vi "Test_IncrementValuePublication_String_ErrorReturned.vi"(8 "error in (no error)":errorcluster, 11 "TestCase in":refnum<class "TestPublicationPolicy.lvclass">) -> (0 "error out":errorcluster, 3 "TestCase out":refnum<class "TestPublicationPolicy.lvclass">)   [LabVIEW 2017, in "TestPublicationPolicy.lvclass"]
uses:
  TestPublicationPolicy.lvclass
  Source/Framework/PublicationPolicy/IncrementValuePublication/IncrementValuePublication.lvclass
  C:/Git/mva-framework/Source/Framework/IMediator/IPublicationPolicy/IPublicationPolicy.lvclass
  Source/Framework/IMediator/IPublicationPolicy/IPublicationPolicy.lvclass
  gpm_packages/@cs/transport/Source/Concrete/NotifierTransport/NotifierTransport.lvclass/NotifierTransport.ctl
  Source/Framework/IMediator/PublishRequest/PublishRequest.lvclass/PublishRequest.ctl
  Source/Framework/IMediator/MutexedPublishRequest/MutexedPublishRequest.lvclass/MutexedPublishRequest.ctl
  Source/Framework/IMediator/PublishRequest/Write Publish Request Data.vi
  gpm_packages/@cs/transport/Source/Concrete/NotifierTransport/NotifierTransport.lvclass
  C:/Git/mva-framework/gpm_packages/@cs/transport/Source/ITransport/ITransport.lvclass
  Source/Framework/IMediator/MutexedPublishRequest/MutexedPublishRequest.lvclass
  C:/Git/mva-framework/Source/Framework/IMediator/PublishRequest/PublishRequest.lvclass
  <vilib>/Utility/error.llb/Error Cluster From Error Code.vi
panel:
  out "Publish Return Error":errorcluster
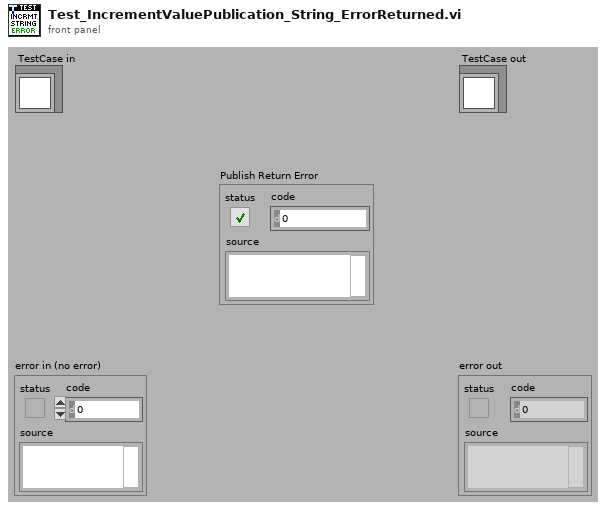
[diagram p1: front panel]
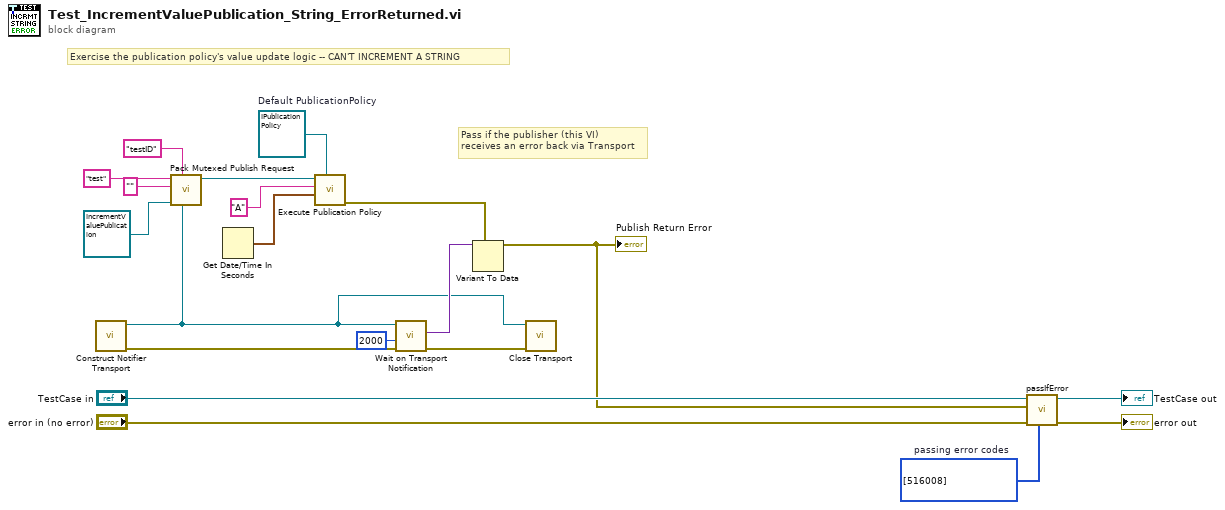
[diagram p0: block diagram]
diagram:
  w3 = i32[] [516008]  # passing error codes
  w12 = refnum<class "IPublicationPolicy.lvclass"> refnum  # Default PublicationPolicy
  # "Pass if the publisher (this VI)\nreceives an error back via Transport"
  # "Exercise the publication policy's value update logic -- CAN'T INCREMENT A STRING"
  n1 = call "Construct Notifier Transport.vi"() -> ("error out"=w8:errorcluster, "NotifierTransport"=w2:refnum<class "NotifierTransport.lvclass">)  [unwired: 10 in]
  n2 = call "Pack Mutexed Publish Request.vi"("Return Error Transport"=w2, "Publisher ID"="testID", "PublicationPolicy"=refnum<class "IncrementValuePublication.lvclass"> refnum ("PublicationPolicy.lvlib:IncrementValuePublication.lvclass"), "Datum Value or Type"="" ("Data to Publish"), "Datum Name"="test") -> ("MutexedPublishRequest Out"=w14:refnum<class "MutexedPublishRequest.lvclass">)  [unwired: 6 in]
  n3 = Get Date/Time In Seconds() -> (seconds since 1Jan1904=w15:timestamp)
  n4 = call-dynamic "Execute Publication Policy.vi"("Default PublicationPolicy"=w12, "Last Publish Time"=w15, "Last Published Value"="A", "MutexedPublishRequest"=w14) -> ("error out (Reject Publication)"=w5:errorcluster)  [unwired: 5 in, 2 out]
  n5 = call "Wait on Transport Notification.vi"("error in (no error)"=w8, "Timeout In ms (-1)"=2000, "NotifierTransport"=w2) -> ("error out"=w1:errorcluster, "Data"=w6:variant)  [unwired: 6 in, 1 out]
  n6 = Variant To Data(type=w5, Variant=w6) -> (data=w4:errorcluster)  [unwired: 1 in, 1 out]
  "Publish Return Error" <- w4
  n7 = call-dynamic "Close Transport.vi"("error in (no error)"=w1, "NotifierTransport"=w2) -> ()  [unwired: 9 in, 1 out]
  n8 = call-dynamic "passIfError.vi"("passing error codes (default = any error code)"=w3, "error in (no error)"="error in (no error)", "error"=w4, "TestCase in"="TestCase in") -> ("error out"=→"error out":errorcluster, "TestCase out"=→"TestCase out":refnum<class "TestPublicationPolicy.lvclass">)  [unwired: 6 in]
